vi "Normalize Point.vi"(1 "point in":cluster{"x":sgl, "y":sgl}) -> (0 "point out":cluster{"x":sgl, "y":sgl})   [LabVIEW 2025]
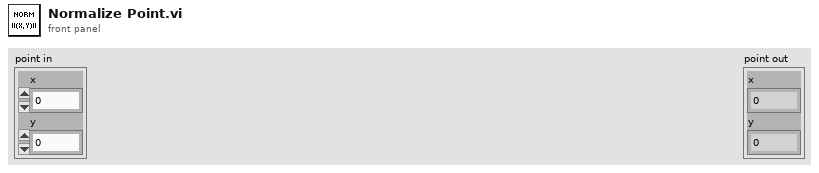
[diagram p1: front panel]
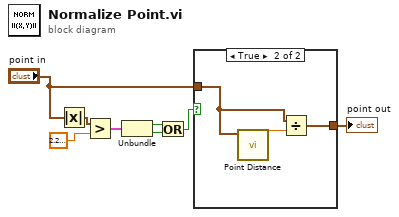
[diagram p0: block diagram]
diagram:
  n1 = Absolute Value(x="point in") -> (abs(x)=w1:cluster{"x":sgl, "y":sgl})
  n2 = Greater?(x=w1, y=2.220446049250313e-16) -> (0:w6:cluster{"x":bool, "y":bool})
  n3 = Unbundle(w6) -> ("x"=w5:bool, "y"=w4:bool)
  n4 = Or(x=w5, y=w4) -> (x .or. y?=w3:bool)
  n5 = case shown="True" w3 {
    tunnel: "point in" -> [_ w10]
    tunnel: [_ w9] -> w8
    frame False {
    }
    frame True {
      n6 = call "Point Distance.vi"("point a"=w10) -> ("dist"=w11:sgl)  [unwired: 10 in]
      n7 = Divide(x=w10, y=w11) -> (x/y=w9:cluster{"x":sgl, "y":sgl})
    }
  }
  "point out" <- w8
